vi "Swerve Wheel.vi"(1 "Wheel":T2(ring)=enum."Front Right", 2 "Inputs":dbl[](array[numeric])=[0.0, -0.10193669212665253, -0.14931439584198622, 0.0, 0.0, 10.75, 15.027058927148719, 10.5], 3 "br offset":dbl(knob)=-6.7034593303000065 scale=-180.0..180.0, 4 "bl offset":dbl(knob)=27.320075486284452 scale=-180.0..180.0, 5 "fr offset":dbl(knob)=31.44769799349993 scale=-180.0..180.0, 6 "fl offset":dbl(knob)=31.73032709235852 scale=-180.0..180.0) -> (0 "Speed":dbl=0.1807923615847232)   [LabVIEW 2016]
uses:
  <vilib>/addons/control/pid/pid.llb/PID (DBL).vi
  <vilib>/addons/control/pid/NI_PID_pid.lvlib
panel:
  in  "PID gains":T1={"proportional gain (Kc)"=0.008, "integral time (Ti, min)"=0.0, "derivative time (Td, min)"=0.1}
  # "Practice Robot Offsets (3-27-17)\n\nFL:  33\nFR: 32\nBL: 30\nBR:  -178"
  # "Gamer Bot Offsets (3/29/17)\n\nFL: -.7\nFR: -165.5\nBL: 98.2\nBR: -66.7"
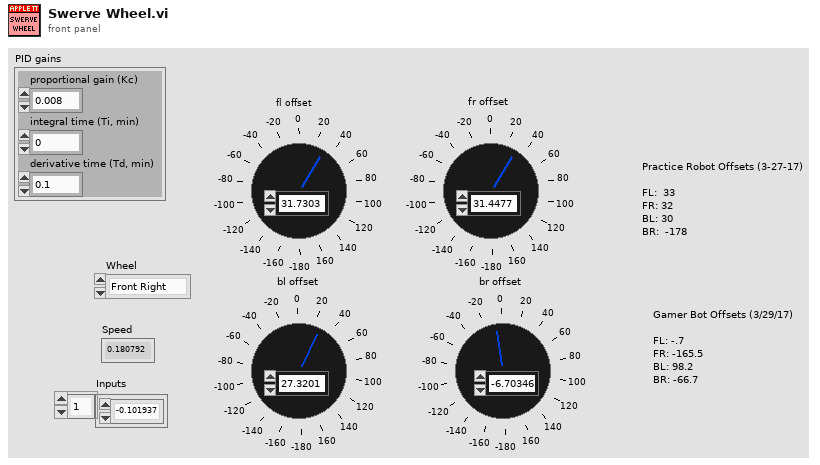
[diagram p1: front panel]
types:
  T1 = cluster{"proportional gain (Kc)":dbl, "integral time (Ti, min)":dbl, "derivative time (Td, min)":dbl}
  T2 = enum16{"Back Left", "Back Right", "Front Left", "Front Right"}
  T3 = enum16{"Z", "Y", "X", "Rot. Point X", "Rot. Point Y", "Width/2", "Max", "Length/2"}
  T4 = enum16{"Z Axis", "Y", "X", "Rot. Point X", "Rot. Point Y", "Width/2", "Max", "Length/2"}
  T5 = typedef "WPI_MotorControlDeviceRef.ctl" = cluster{"DeviceStatus":errorcluster, "Type":T6, "PWM":cluster{"PWM Channel":T7, "DeadBand":T8}, "CAN":cluster{"Device Number":u8, "SetOutput VI Ref":variant, "GetOutput VI Ref":variant, "Enable VI Ref":variant, "Disable VI Ref":variant, "Data":variant}, "Invert":bool}
  T6 = typedef "WPI_MotorControlType.ctl" = enum16{"PWM", "CAN"}
  T7 = typedef "FPGA_DIOPWMChannel.ctl" = enum8{"PWM 0", "PWM 1", "PWM 2", "PWM 3", "PWM 4", "PWM 5", "PWM 6", "PWM 7", "PWM 8", "PWM 9", "PWM MXP 0", "PWM MXP 1", "PWM MXP 2", "PWM MXP 3", "PWM MXP 4", "PWM MXP 5", "PWM MXP 6", "PWM MXP 7", "PWM MXP 8", "PWM MXP 9", "Invalid"}
  T8 = typedef "WPI_PWMDeadband.ctl" = cluster{"Name":string, "maxPositivePwm":i32, "minPositivePwm":i32, "centerPwm":i32, "maxNegativePwm":i32, "minNegativePwm":i32, "angularRange":u16}
  T9 = typedef "WPI_CANTalonSRX_GlobalStatus.ctl" = cluster{"Applied Throttle":dbl, "Module Enabled":bool, "CAN Error":errorcluster, "Closed Loop Error":dbl, "Forward Limit Switch Closed":bool, "Reverse Limit Switch Closed":bool, "Sensor Position":dbl, "Sensor Velocity":dbl, "Current":dbl, "Sticky Fault - Over Temp":bool, "Sticky Fault - Under Voltage":bool, "Sticky Fault - Forward Limit":bool, "Sticky Fault - Reverse Limit":bool, "Sticky Fault - Forward Soft Limit":bool, "Sticky Fault - Reverse Soft Limit":bool, "Brake is Enabled":bool, "Encoder Position":dbl, "Encoder Velocity":dbl, "Encoder Index Count":dbl, "Encoder A Pin State":bool, "Encoder B Pin State":bool, "Encoder Index Pin State":bool, "Analog In":dbl, "Analog In Velocity":dbl, "Temperature (C)":dbl, "Battery Voltage":dbl, "Control 5 Is Supported":bool, "Current Profile Slot Select":dbl, "Pos Div 8":bool, "Vel Div 4":bool, "Pulse Width Position":i32, "Pulse Width Velocity":i32, "Pulse Width Rise To Rise (us)":i32, "Pulse Width Rise To Fall (us)":i32, "Mot Prof Active Is Under Run":bool, "Mot Prof Active Has Under Run":bool, "Mot Prof Active Is Last":bool, "Mot Prof Active Velocity Only":bool, "Mot Prof Active Is Valid":bool, "Mot Prof Buffer Is Full":bool, "Mot Prof Active Profile Slot Select":i32, "Mot Prof NextID":i32, "Mot Prof Count":i32, "Mot Prof Active Velocity":dbl, "Mot Prof Active Position":dbl, "Mot Prof Output Enable":i32, "UsageFrame":u32, "Motion Magic Active Trajectory":cluster{"Velocity":dbl, "Position":dbl}}
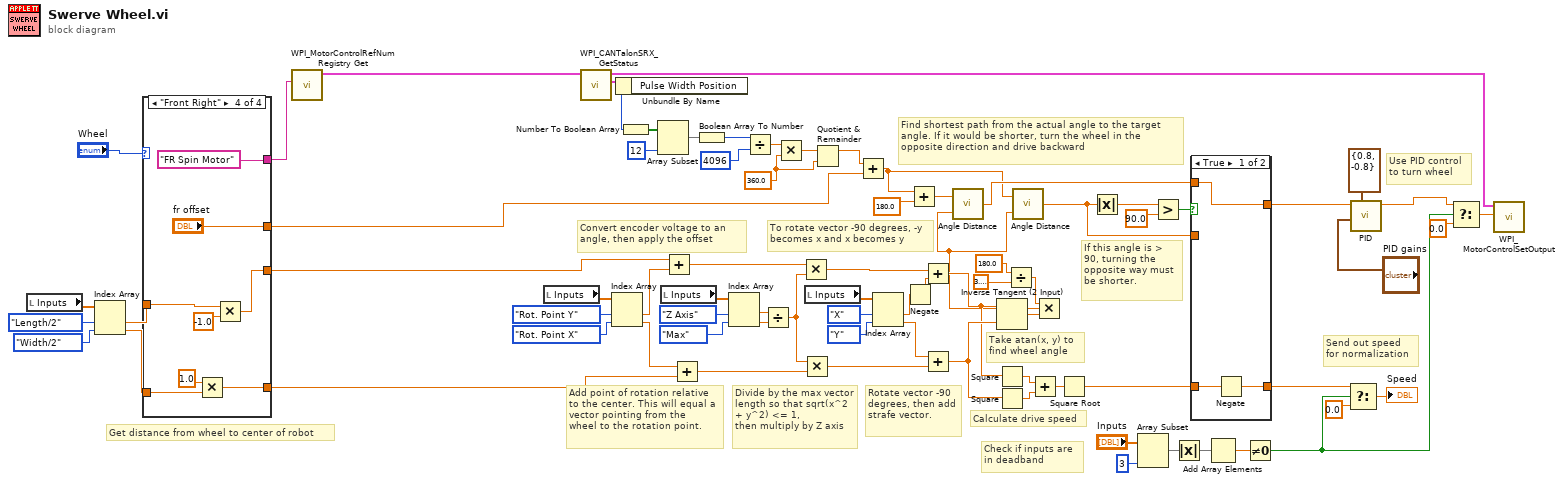
[diagram p0: block diagram]
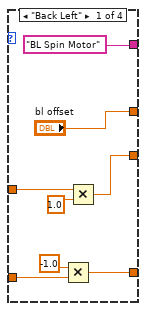
[diagram p3: hidden frame]
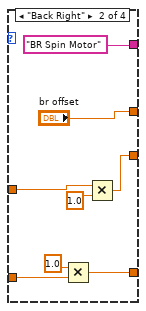
[diagram p4: hidden frame]
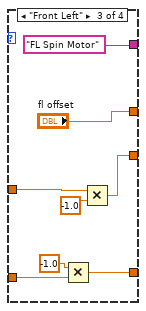
[diagram p5: hidden frame]
diagram:
  w2 = 360.0 ("y")
  # "To rotate vector -90 degrees, -y becomes x and x becomes y"
  # "Divide by the max vector length so that sqrt(x^2 + y^2) <= 1,\nthen multiply by Z axis"
  # "Add point of rotation relative to the center. This will equal a vector pointing from the\nwheel to the rotation point."
  # "Send out speed\nfor normalization"
  # "Check if inputs are\nin deadband"
  # "Convert encoder voltage to an angle, then apply the offset"
  # "If this angle is > 90, turning the opposite way must be shorter."
  # "Use PID control\nto turn wheel"
  # "Find shortest path from the actual angle to the target angle. If it would be shorter, turn the wheel in the opposite direction and drive backward"
  # "Take atan(x, y) to find wheel angle"
  # "Calculate drive speed"
  # "Rotate vector -90 degrees, then add strafe vector."
  # "Get distance from wheel to center of robot"
  n1 = local read "Inputs"() -> (w28:dbl[])
  n2 = Index Array(array=w28, index #1=T3."Length/2", index #2=T3."Width/2") -> (element #1=w26:dbl, element #2=w25:dbl)
  n3 = case shown="\"Front Right\"" "Wheel" {
    tunnel: ["BL Spin Motor" "BR Spin Motor" "FL Spin Motor" "FR Spin Motor"] -> w64
    tunnel: ["bl offset" "br offset" "fl offset" "fr offset"] -> w6
    tunnel: w26 -> [w84 w92 w100 w108]
    tunnel: w25 -> [w82 w90 w99 w106]
    tunnel: [w81 w89 w98 w105] -> w51
    tunnel: [w80 w88 w97 w104] -> w47
    frame "Back Left" {
      n4 = Multiply(x=-1.0 ("y"), y=w82) -> (x*y=w80:dbl)
      n5 = Multiply(x=w84, y=1.0) -> (x*y=w81:dbl)
    }
    frame "Back Right" {
      n6 = Multiply(x=1.0 ("y"), y=w90) -> (x*y=w88:dbl)
      n7 = Multiply(x=w92, y=1.0) -> (x*y=w89:dbl)
    }
    frame "Front Left" {
      n8 = Multiply(x=-1.0 ("y"), y=w99) -> (x*y=w97:dbl)
      n9 = Multiply(x=w100, y=-1.0) -> (x*y=w98:dbl)
    }
    frame "Front Right" {
      n10 = Multiply(x=1.0 ("y"), y=w106) -> (x*y=w104:dbl)
      n11 = Multiply(x=w108, y=-1.0) -> (x*y=w105:dbl)
    }
  }
  n12 = call <vilib>:"WPI_MotorControlRefNum Registry Get.vi"("refnum name"=w64) -> ("MotorControlDevRef"=w5:T5)  [unwired: 9 in, 1 out]
  n13 = local read "Inputs"() -> (w49:dbl[])
  n14 = call <vilib>:"WPI_CANTalonSRX_GetStatus.vi"("CAN Talon SRX Ref"=w5) -> ("Talon SRX Status"=w15:T9, "CAN Talon SRX Ref"=w4:T5)  [unwired: 8 in, 1 out]
  n15 = Index Array(array=w49, index #1=T3."Rot. Point Y", index #2=T3."Rot. Point X") -> (element #1=w45:dbl, element #2=w46:dbl)
  n16 = Unbundle By Name(w15) -> ("Pulse Width Position"=w11:i32)
  n17 = Number To Boolean Array(number=w11) -> (Boolean array=w13:bool[])
  n18 = Array Subset(array=w13, length=12 ("index")) -> (w12:bool[])  [unwired: 1 in]
  n19 = local read "Inputs"() -> (w43:dbl[])
  n20 = Add(x=w51, y=w45) -> (x+y=w23:dbl)
  n21 = Add(x=w46, y=w47) -> (x+y=w39:dbl)
  n22 = Boolean Array To Number(Boolean array=w12) -> (number=w10:u32)
  n23 = Index Array(array=w43, index #1=T4."Z Axis", index #2=T3."Max") -> (element #1=w40:dbl, element #2=w41:dbl)
  n24 = Divide(x=w10, y=u32 4096) -> (x/y=w8:dbl)
  n25 = Divide(x=w40, y=w41) -> (x/y=w38:dbl)
  n26 = Multiply(x=w8, y=w2) -> (x*y=w3:dbl)
  n27 = Multiply(x=w23, y=w38) -> (x*y=w18:dbl)
  n28 = Multiply(x=w38, y=w39) -> (x*y=w33:dbl)
  n29 = local read "Inputs"() -> (w36:dbl[])
  n30 = Quotient & Remainder(x=w3, y=w2) -> (x-y*floor(x/y)=w1:dbl)  [unwired: 1 out]
  n31 = Add(x=w1, y=w6) -> (x+y=w7:dbl)
  n32 = Index Array(array=w36, index #1=T3."X", index #2=T3."Y") -> (element #1=w16:dbl, element #2=w32:dbl)
  n33 = Negate(x=w16) -> (-x=w17:dbl)
  n34 = Add(x=w7, y=180.0 ("f")) -> (x+y=w59:dbl)
  n35 = Add(x=w18, y=w17) -> (x+y=w30:dbl)
  n36 = Add(x=w32, y=w33) -> (x+y=w31:dbl)
  n37 = Inverse Tangent (2 Input)(1:w31, 2:w30) -> (0:w75:dbl)
  n38 = Square(x=w30) -> (x^2=w34:dbl)
  n39 = Square(x=w31) -> (x^2=w74:dbl)
  n40 = Divide(x=180.0 ("y"), y=3.141592653589793) -> (x/y=w72:dbl)
  n41 = Add(x=w34, y=w74) -> (x+y=w73:dbl)
  n42 = Multiply(x=w72, y=w75) -> (x*y=w24:dbl)
  n43 = call "Angle Distance.vi"("target angle"=w24, "current angle"=w59) -> ("distance"=w21:dbl)
  n44 = call "Angle Distance.vi"("target angle"=w24, "current angle"=w7) -> ("distance"=w66:dbl)
  n45 = Square Root(x=w73) -> (sqrt(x)=w65:dbl)
  n46 = Absolute Value(x=w66) -> (abs(x)=w67:dbl)
  n47 = Array Subset(array="Inputs", length=3) -> (w58:dbl[])  [unwired: 1 in]
  n48 = Greater?(x=w67, y=90.0) -> (0:w54:bool)
  n49 = Absolute Value(x=w58) -> (abs(x)=w52:dbl[])
  n50 = case shown="True" w54 {
    tunnel: w21 -> [w111 _]
    tunnel: w66 -> [_ w115]
    tunnel: [w112 w114] -> w57
    tunnel: w65 -> [w113 w114]
    tunnel: [w111 w115] -> w20
    frame True {
      n51 = Negate(x=w113) -> (-x=w112:dbl)
    }
    frame False {
    }
  }
  n52 = Add Array Elements(numeric array=w52) -> (sum=w76:dbl)
  n53 = Not Equal To 0?(x=w76) -> (x != 0?=w53:bool)
  n54 = Select(t=w57, s=w53, f=0.0) -> (s? t:f=→"Speed":dbl)
  n55 = call-poly <vilib>:"PID.vi"("output range"=cluster{"output high":dbl, "output low":dbl} {"output high"=0.8, "output low"=-0.8}, "PID gains"="PID gains", "setpoint"=w20) -> ("output"=w19:dbl)  [unwired: 7 in, 1 out]
  n56 = Select(t=w19, s=w53, f=0.0) -> (s? t:f=w61:dbl)
  n57 = call <vilib>:"WPI_MotorControlSetOutput.vi"("Output"=w61, "MotorControlDevRef"=w4) -> ()  [unwired: 7 in, 3 out]
